vi "writeTimingXML.vi"(8 "error in (no error)":errorcluster, 10 "NativeXML in":refnum<class "NativeXML.lvclass">, 11 "PixelflySettings in":refnum<class "PixelflySettings.lvclass">) -> (0 "error out":errorcluster, 2 "NativeXML out":refnum<class "NativeXML.lvclass">, 3 "PixelflySettings out":refnum<class "PixelflySettings.lvclass">)   [LabVIEW 2009, in "Tools.lvlib" / "Settings.lvlib" / "PixelflySettings.lvclass"]
uses:
  PixelflySettings.lvclass
  NativeXML/NativeXML.lvclass
  PixelflySettings.lvclass/PixelflySettings.ctl
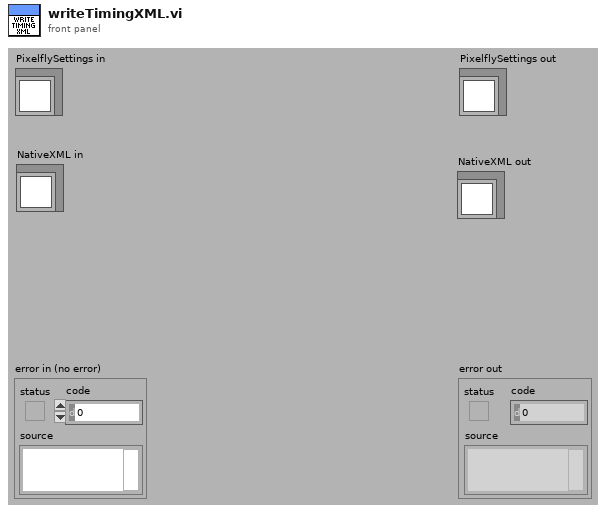
[diagram p1: front panel]
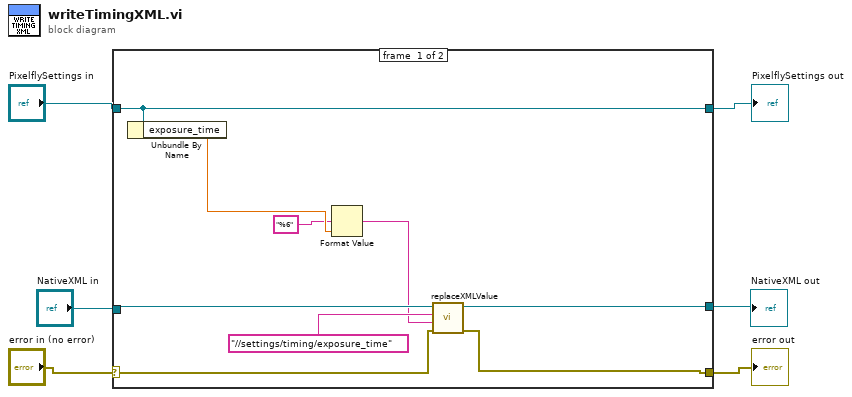
[diagram p0: block diagram]
diagram:
  n1 = case shown="No Error" "error in (no error)" {
    selector: "error in (no error)" -> [w11 w18]
    tunnel: [w10 w18] -> w4
    tunnel: [w15 w17] -> w5
    tunnel: "PixelflySettings in" -> [w15 w17]
    tunnel: "NativeXML in" -> [w14 w16]
    tunnel: [w13 w16] -> w3
    frame #0 {
      n2 = Unbundle By Name(w15) -> ("exposure_time"=w9:dbl)
      n3 = Format Value(format string="%6", value (0)=w9) -> (output string=w7:string)  [unwired: 1 in]
      n4 = call "replaceXMLValue.vi"("error in (no error)"=w11, "value"=w7, "replace in"="//settings/timing/exposure_time", "NativeXML in"=w14) -> ("error out"=w10:errorcluster, "NativeXML out"=w13:refnum<class "NativeXML.lvclass">)  [unwired: 6 in]
    }
    frame #1 {
    }
  }
  "error out" <- w4
  "PixelflySettings out" <- w5
  "NativeXML out" <- w3
